vi "Data_Process_1.vi"(5 "Offset_Error":dbl[](array[numeric]), 6 "ADC+CH":string[](array[string]), 7 "Gain_Error":dbl[](array[numeric]), 8 "ACQPS":string, 9 "Std_Deviation":dbl[][](array[numeric]), 10 "Mean":dbl[][](array[numeric]), 11 "Vin_Measured":dbl[][](array[numeric])) -> (0 "OFF+GAIN":string[][](array[string]), 2 "output array":string[][](array[string]))   [LabVIEW 2019]
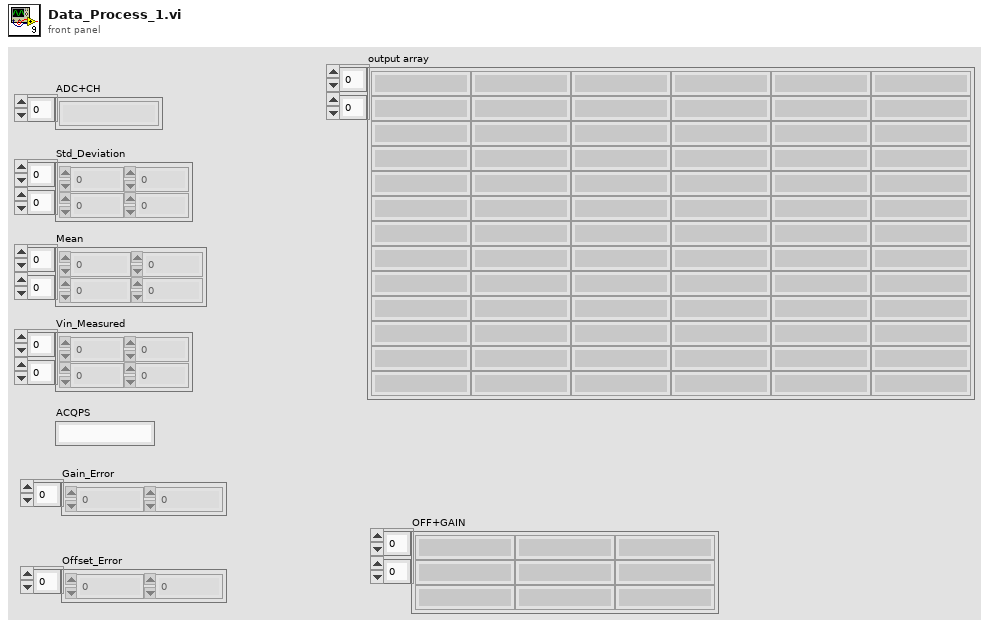
[diagram p1: front panel]
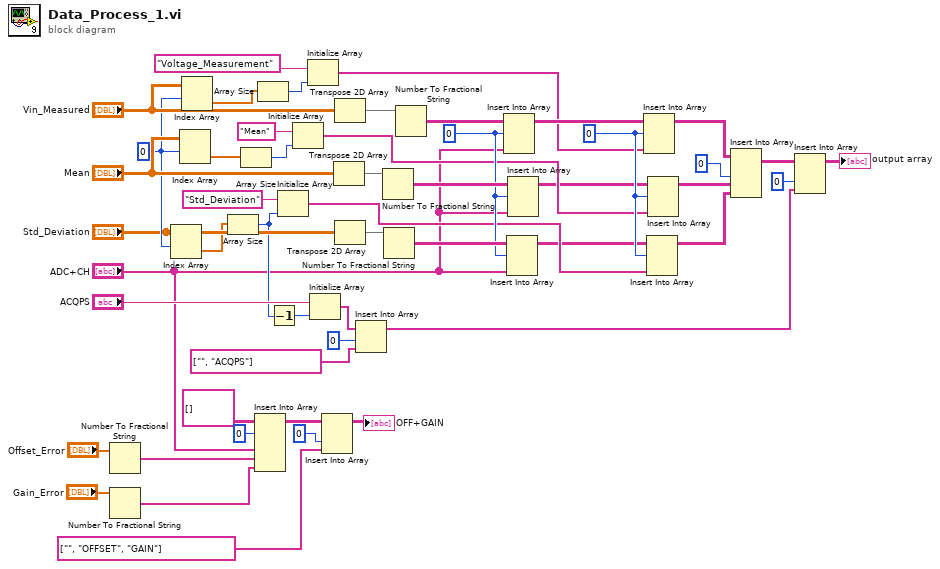
[diagram p0: block diagram]
diagram:
  w31 = 0 ("index (row)")
  w37 = 0 ("index (row)")
  w45 = 0 ("index (row)")
  n1 = Number To Fractional String(number="Offset_Error") -> (F-format string=w7:string[])  [unwired: 3 in]
  n2 = Number To Fractional String(number="Gain_Error") -> (F-format string=w3:string[])  [unwired: 3 in]
  n3 = Index Array(array="Std_Deviation", index (row)=w37) -> (element=w34:dbl[])  [unwired: 1 in]
  n4 = Index Array(array="Mean", index (row)=w37) -> (element=w33:dbl[])  [unwired: 1 in]
  n5 = Index Array(array="Vin_Measured", index (row)=w37) -> (element=w32:dbl[])  [unwired: 1 in]
  n6 = Array Size(array=w34) -> (size(s)=w18:i32)
  n7 = Array Size(array=w33) -> (size(s)=w35:i32)
  n8 = Insert Into Array(array=string[][] [], index (row)=0, new element #1="ADC+CH", new element #2=w7, new element #3=w3) -> (w5:string[][])  [unwired: 1 in]
  n9 = Array Size(array=w32) -> (size(s)=w40:i32)
  n10 = Decrement(x=w18) -> (x-1=w17:i32)
  n11 = Initialize Array("Std_Deviation", w18) -> (w23:string[])
  n12 = Initialize Array("Mean", w35) -> (w27:string[])
  n13 = Initialize Array("Voltage_Measurement", w40) -> (w28:string[])
  n14 = Initialize Array("ACQPS", w17) -> (w19:string[])
  n15 = Insert Into Array(array=w5, index (col)=0 ("index (row)"), new element=string[] ["", "OFFSET", "GAIN"]) -> (→"OFF+GAIN":string[][])  [unwired: 1 in]
  n16 = Transpose 2D Array(2D array="Mean") -> (transposed array=w49:dbl[][])
  n17 = Transpose 2D Array(2D array="Vin_Measured") -> (transposed array=w48:dbl[][])
  n18 = Transpose 2D Array(2D array="Std_Deviation") -> (transposed array=w50:dbl[][])
  n19 = Insert Into Array(array=w19, index=0, new element=string[] ["", "ACQPS"]) -> (w15:string[])
  n20 = Number To Fractional String(number=w49) -> (F-format string=w46:string[][])  [unwired: 3 in]
  n21 = Number To Fractional String(number=w50) -> (F-format string=w47:string[][])  [unwired: 3 in]
  n22 = Number To Fractional String(number=w48) -> (F-format string=w51:string[][])  [unwired: 3 in]
  n23 = Insert Into Array(array=w51, index (row)=w45, new element="ADC+CH") -> (w30:string[][])  [unwired: 1 in]
  n24 = Insert Into Array(array=w47, index (row)=w45, new element="ADC+CH") -> (w22:string[][])  [unwired: 1 in]
  n25 = Insert Into Array(array=w46, index (row)=w45, new element="ADC+CH") -> (w24:string[][])  [unwired: 1 in]
  n26 = Insert Into Array(array=w30, index (row)=w31, new element=w28) -> (w29:string[][])  [unwired: 1 in]
  n27 = Insert Into Array(array=w22, index (row)=w31, new element=w23) -> (w26:string[][])  [unwired: 1 in]
  n28 = Insert Into Array(array=w24, index (row)=w31, new element=w27) -> (w25:string[][])  [unwired: 1 in]
  n29 = Insert Into Array(array=w29, index (col)=0 ("disabled index (col)"), new element #1=w25, new element #2=w26) -> (w20:string[][])  [unwired: 1 in]
  n30 = Insert Into Array(array=w20, index (col)=0 ("disabled index (col)"), new element=w15) -> (→"output array":string[][])  [unwired: 1 in]
